vi "arrayWaveformGenerator.vi"(8 "error in (no error)":errorcluster, 11 "signal generation parameters":T1(array[cluster])=[{"signal type"=enum."Square Wave", "frequency"=100.0, "amplitude"=1.0, "phase"=0.0, "offset"=0.0, "duty cycle (%)"=50.0, "reset signal"=FALSE, "sampling info"={"Fs"=1000.0, "#s"=100.0}}, {"signal type"=enum."Triangle Wave", "frequency"=80.0, "amplitude"=0.0, "phase"=0.0, "offset"=0.0, "duty cycle (%)"=0.0, "reset signal"=FALSE, "sampling info"={"Fs"=1000.0, "#s"=100.0}}] {"sampling info"."#s" format="%#.6g"; "sampling info"."Fs" format="%0.2p"; "duty cycle (%)" format="%#.6g"; "offset" format="%#.6g"; "phase" format="%#.6g"; "amplitude" format="%#.6g"; "frequency" format="%#.6g"}) -> (0 "error out":errorcluster, 1 "phase out":dbl[](array[numeric]), 2 "signal out":waveform(dbl)[](array[waveform]))   [LabVIEW 2023]
doc: "This VI creates an output waveform that is one of the common signal types: Sine wave, Triangle, Sawtooth, or Square wave. This VI remembers the timestamp of the previous waveform generated and continues to increment the timestamp from that point. It takes as inputs the type of waveform, number of samples, phase, and frequency."
uses:
  <vilib>/Analysis/NI_AALBase.lvlib
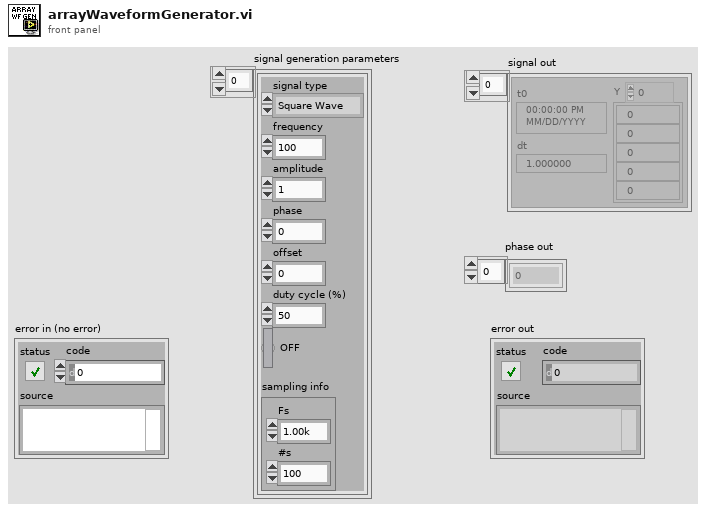
[diagram p1: front panel]
types:
  T1 = cluster{"signal type":enum16{"Sine Wave", "Triangle Wave", "Square Wave", "Sawtooth Wave"}, "frequency":dbl, "amplitude":dbl, "phase":dbl, "offset":dbl, "duty cycle (%)":dbl, "reset signal":bool, "sampling info":cluster{"Fs":dbl, "#s":dbl}}[]
  T2 = enum16{"Sine Wave", "Triangle Wave", "Square Wave", "Sawtooth Wave"}
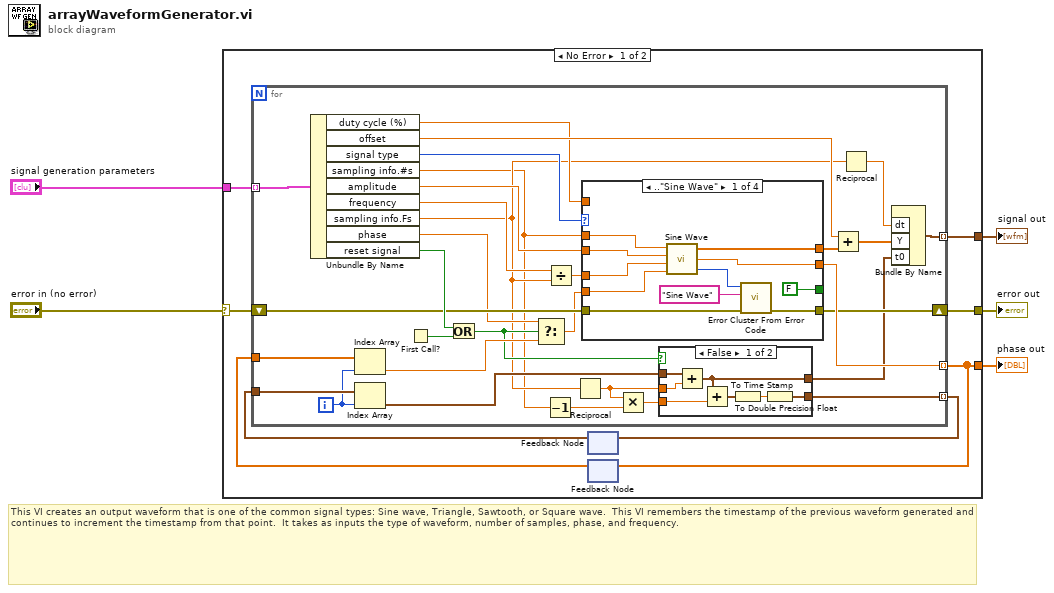
[diagram p0: block diagram]
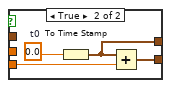
[diagram p2: hidden frame]
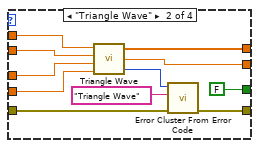
[diagram p3: hidden frame]
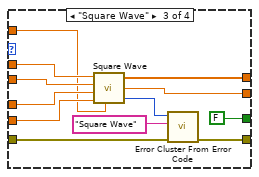
[diagram p4: hidden frame]
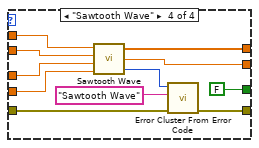
[diagram p5: hidden frame]
diagram:
  # "This VI creates an output waveform that is one of the common signal types: Sine wave, Triangle, Sawtooth, or Square wave.  This VI remembers the timestamp of the previous waveform generated and continues to increment the timestamp from that point.  It takes as inputs the type of waveform, number of samples, phase, and frequency."
  n1 = case shown="No Error" "error in (no error)" {
    selector: "error in (no error)" -> [w6 w101]
    tunnel: [w10 _] -> w1
    tunnel: [w11 w101] -> w2
    tunnel: [w13 _] -> w4
    tunnel: "signal generation parameters" -> [w12 _]
    frame No Error {
      n2 = feedback #1() -> (w7:timestamp[])  [unwired: 1 in]
      n3 = feedback #2() -> (w9:dbl[])  [unwired: 1 in]
      n4 = for {
        tunnel: w9 -> [w28]
        tunnel: [w14] -> w8 mode=indexing
        tunnel: w7 -> [w30]
        tunnel: [w40] -> w10 mode=indexing
        tunnel: [w38] -> w13 mode=indexing
        tunnel: w12 -> [w37] mode=indexing
        shift-right: [w39] -> w11
        shift-left: w6 -> [w27]
        i -> [w29]
        n5 = Unbundle By Name(w37) -> ("duty cycle (%)"=w31:dbl, "offset"=w32:dbl, "signal type"=w33:T2, "sampling info.#s"=w16:dbl, "amplitude"=w34:dbl, "frequency"=w35:dbl, "sampling info.Fs"=w18:dbl, "phase"=w25:dbl, "reset signal"=w36:bool)
        n6 = Index Array(array=w28, index=w29) -> (element=w24:dbl)
        n7 = Index Array(array=w30, index=w29) -> (element=w20:timestamp)
        n8 = First Call?() -> (First Call?: T/F=w26:bool)
        n9 = Or(x=w36, y=w26) -> (x .or. y?=w21:bool)
        n10 = Select(t=w25, s=w21, f=w24) -> (s? t:f=w23:dbl)
        n11 = Decrement(x=w16) -> (x-1=w22:dbl)
        n12 = Divide(x=w35, y=w18) -> (x/y=w43:dbl)
        n13 = Reciprocal(x=w18) -> (1/x=w15:dbl)
        n14 = case shown="..\"Sine Wave\"" w33 {
          tunnel: w43 -> [w66 w77 w89 w100]
          tunnel: w34 -> [w65 w76 w88 w99]
          tunnel: w16 -> [w64 w75 w87 w98]
          tunnel: w23 -> [w63 w74 w86 w97]
          tunnel: [w62 w73 w85 w96] -> w40
          tunnel: [w61 w72 w84 w95] -> w42
          tunnel: [w56 w69 w81 w92] -> w39
          tunnel: [FALSE FALSE FALSE FALSE] -> _
          tunnel: w31 -> [_ _ w78 _]
          tunnel: w27 -> [w57 w67 w79 w90]
          frame .."Sine Wave" {
            n15 = call <vilib>:"Sine Wave.vi"("samples"=w64, "amplitude"=w65, "frequency"=w66, "phase in"=w63) -> ("sine wave"=w61:dbl[], "phase out"=w62:dbl, "error"=w59:i32)  [unwired: 1 in]
            n16 = call <vilib>:"Error Cluster From Error Code.vi"("error in (no error)"=w57, "error message (\"\")"="Sine Wave" ("subVI Name"), "error code (0)"=w59) -> ("error out"=w56:errorcluster)  [unwired: 6 in]
          }
          frame "Triangle Wave" {
            n17 = call <vilib>:"Triangle Wave.vi"("samples"=w75, "amplitude"=w76, "frequency"=w77, "phase in"=w74) -> ("triangle wave"=w72:dbl[], "phase out"=w73:dbl, "error"=w71:i32)  [unwired: 1 in]
            n18 = call <vilib>:"Error Cluster From Error Code.vi"("error in (no error)"=w67, "error message (\"\")"="Triangle Wave" ("subVI Name"), "error code (0)"=w71) -> ("error out"=w69:errorcluster)  [unwired: 6 in]
          }
          frame "Square Wave" {
            n19 = call <vilib>:"Square Wave.vi"("samples"=w87, "amplitude"=w88, "frequency"=w89, "duty cycle (%)"=w78, "phase in"=w86) -> ("square wave"=w84:dbl[], "phase out"=w85:dbl, "error"=w83:i32)  [unwired: 1 in]
            n20 = call <vilib>:"Error Cluster From Error Code.vi"("error in (no error)"=w79, "error message (\"\")"="Square Wave" ("subVI Name"), "error code (0)"=w83) -> ("error out"=w81:errorcluster)  [unwired: 6 in]
          }
          frame "Sawtooth Wave" {
            n21 = call <vilib>:"Sawtooth Wave.vi"("samples"=w98, "amplitude"=w99, "frequency"=w100, "phase in"=w97) -> ("sawtooth wave"=w95:dbl[], "phase out"=w96:dbl, "error"=w94:i32)  [unwired: 1 in]
            n22 = call <vilib>:"Error Cluster From Error Code.vi"("error in (no error)"=w90, "error message (\"\")"="Sawtooth Wave" ("subVI Name"), "error code (0)"=w94) -> ("error out"=w92:errorcluster)  [unwired: 6 in]
          }
        }
        n23 = Multiply(x=w15, y=w22) -> (x*y=w17:dbl)
        n24 = case shown="False" w21 {
          tunnel: w20 -> [w51 _]
          tunnel: [w49 w55] -> w19
          tunnel: w15 -> [w50 _]
          tunnel: w17 -> [w48 w54]
          tunnel: [w45 w53] -> w14
          frame False {
            n25 = Add(x=w51, y=w50) -> (x+y=w49:timestamp)
            n26 = Add(x=w49, y=w48) -> (x+y=w47:timestamp)
            n27 = To Double Precision Float(number=w47) -> (double precision float=w46:dbl)
            n28 = To Time Stamp(1:w46) -> (0:w45:timestamp)
          }
          frame True {
            w52 = 0.0  # t0
            n29 = To Time Stamp(1:w52) -> (0:w55:timestamp)
            n30 = Add(x=w55, y=w54) -> (x+y=w53:timestamp)
          }
        }
        n31 = Add(x=w32, y=w42) -> (x+y=w41:dbl[])
        n32 = Reciprocal(x=w18) -> (1/x=w44:dbl)
        n33 = Bundle By Name("dt"=w44, "Y"=w41, "t0"=w19) -> (w38:waveform(dbl))  [unwired: 1 in]
      }
      n34 = feedback-in #1(w8) -> ()
      n35 = feedback-in #2(w10) -> ()
    }
    frame Error {
    }
  }
  "error out" <- w2
  "signal out" <- w4
  "phase out" <- w1
